vi "LuaTo.vi"(6 "Index":i32, 7 "L In":u64, 8 "Lua Dll":path) -> (0 "String":string, 1 "Variant":variant, 2 "Number":dbl, 3 "Boolean":bool, 4 "L Out":u64, 5 "Pointer":u64)   [LabVIEW 2014]
uses:
  LabVIEW.exe
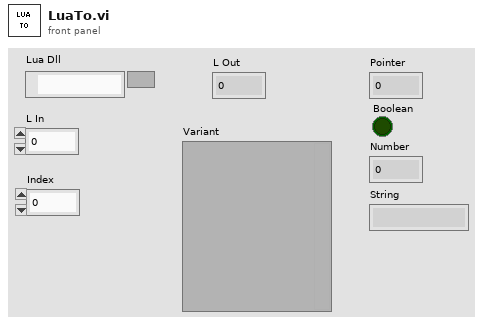
[diagram p1: front panel]
types:
  T1 = enum16{"nil", "boolean", "lightuserdata", "number", "string", "table", "function", "userdata", "thread"}
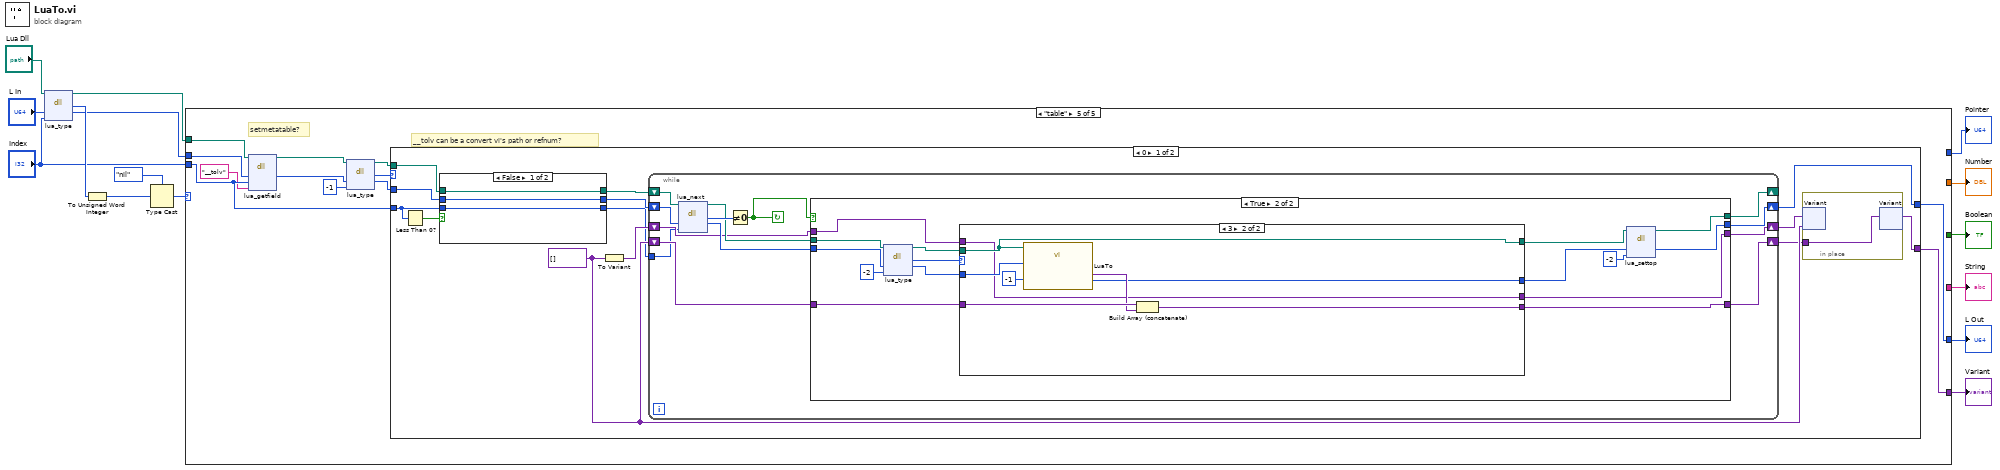
[diagram p0: block diagram]
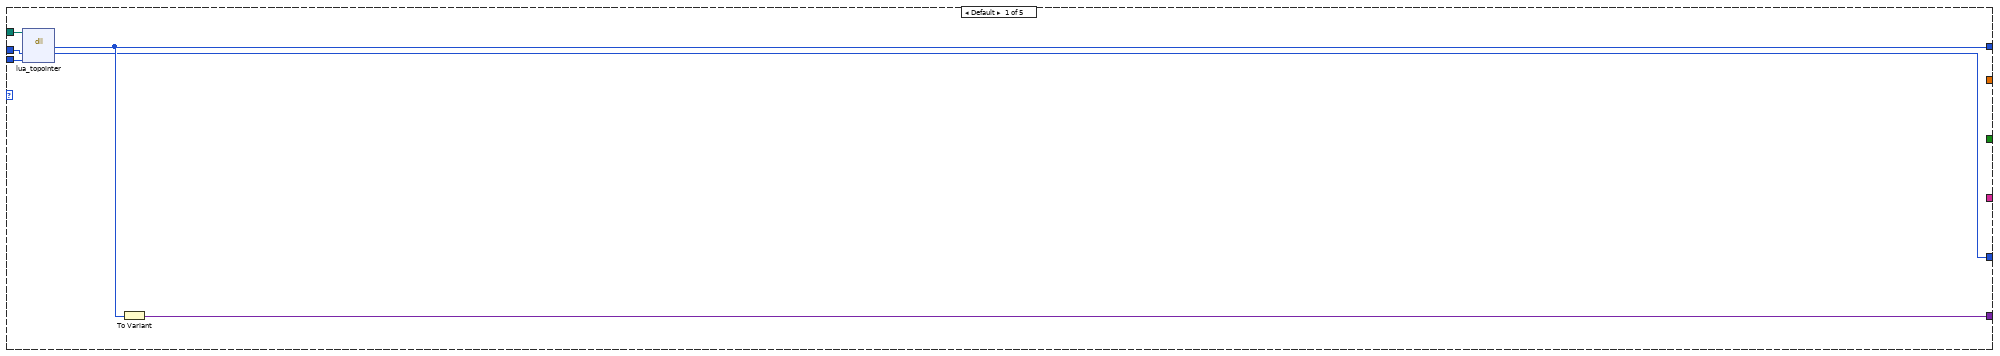
[diagram p2: hidden frame]
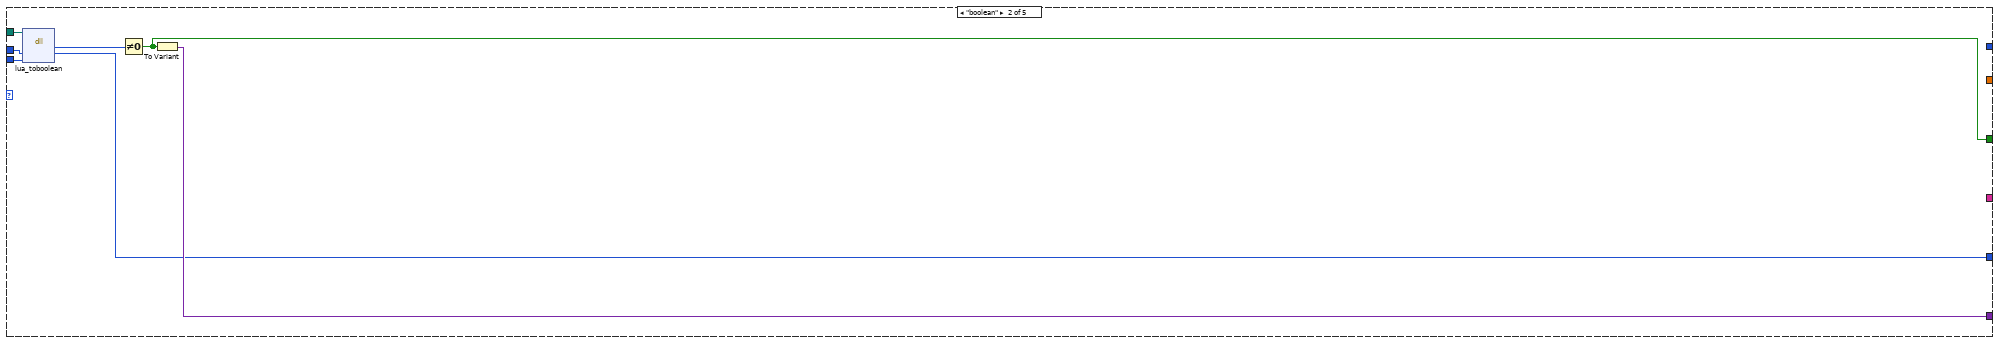
[diagram p3: hidden frame]
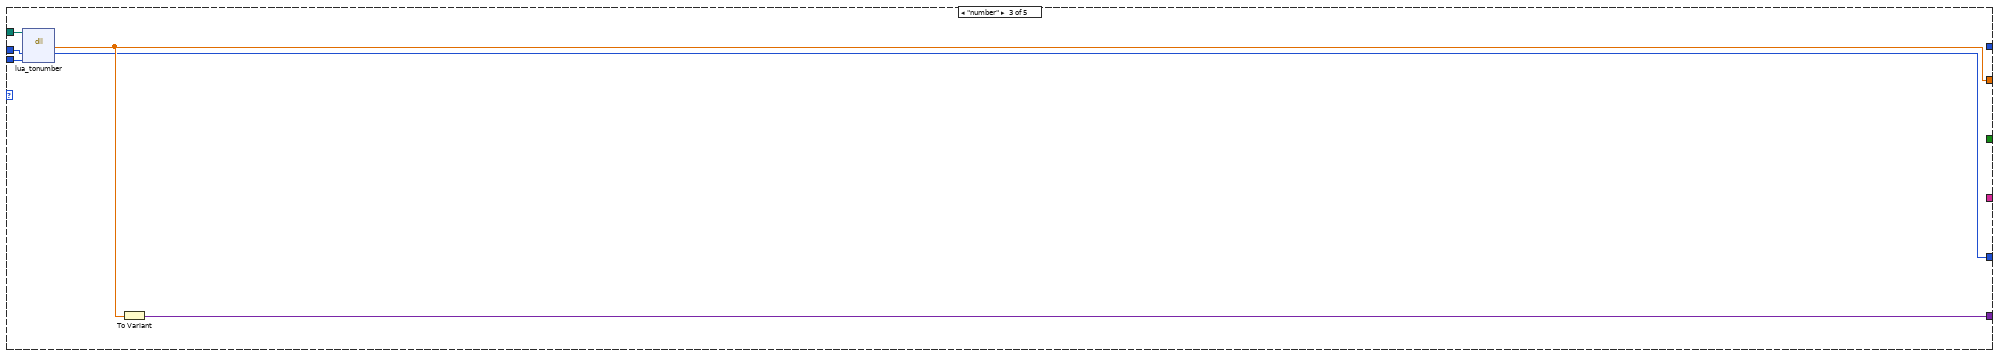
[diagram p4: hidden frame]
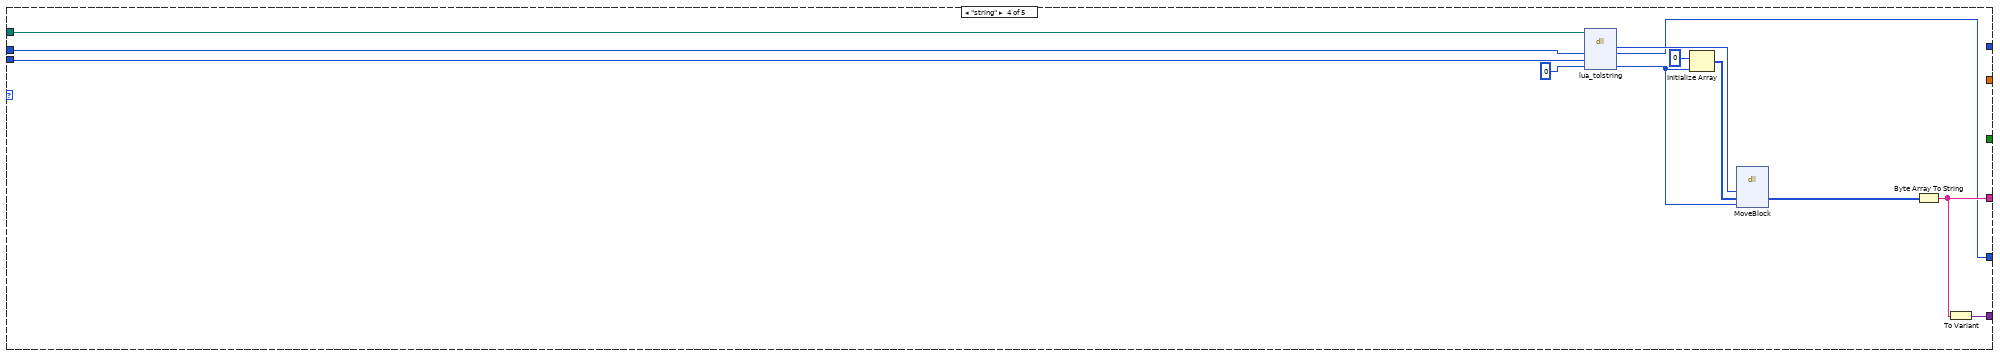
[diagram p5: hidden frame]
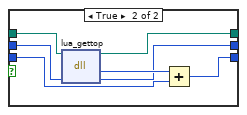
[diagram p6: hidden frame]
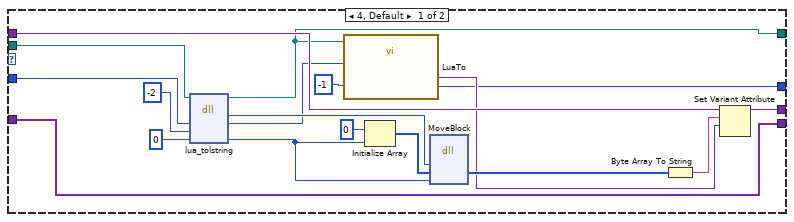
[diagram p8: hidden frame]
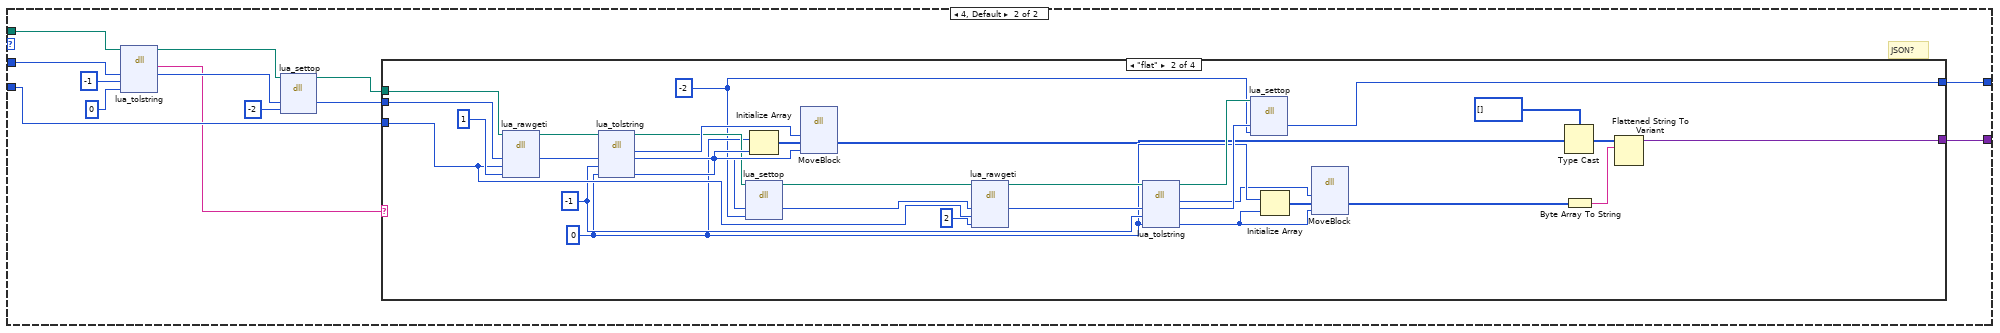
[diagram p9: hidden frame]
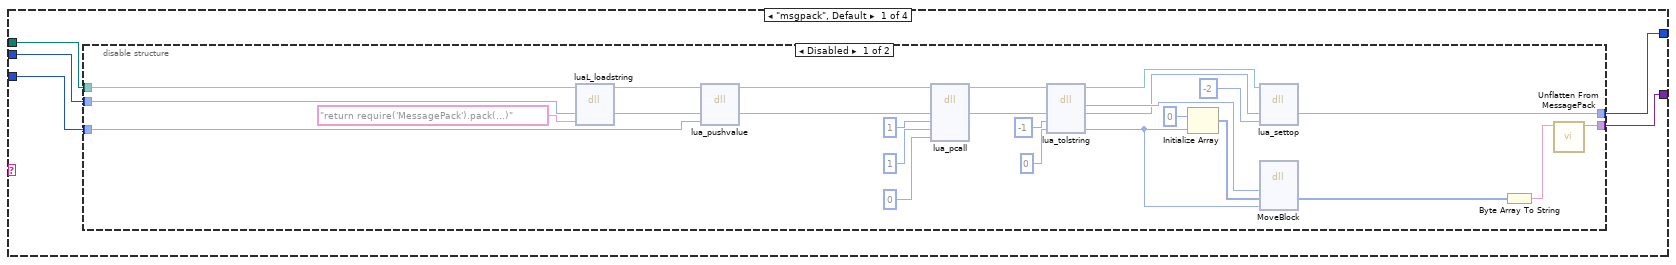
[diagram p10: hidden frame]
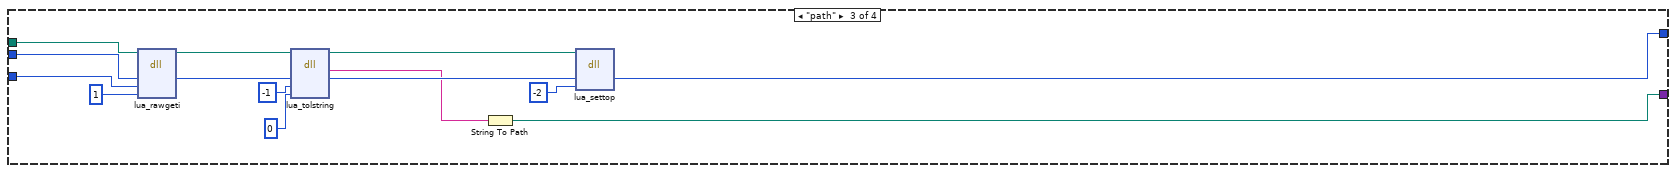
[diagram p12: hidden frame]
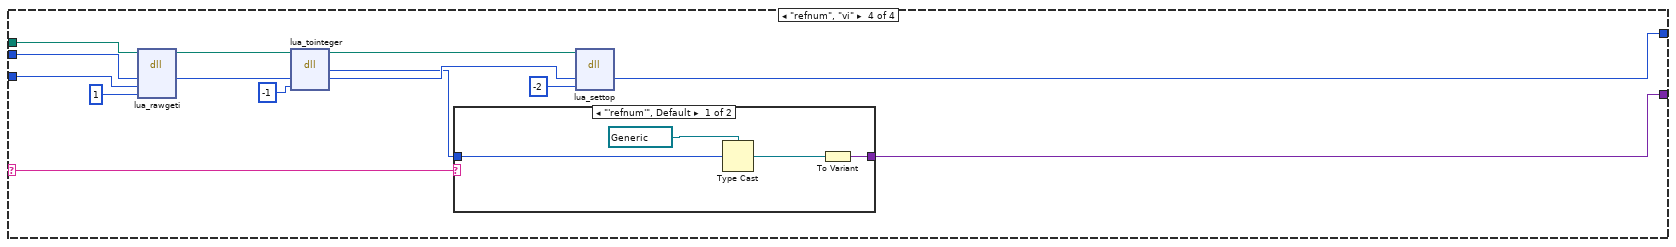
[diagram p13: hidden frame]
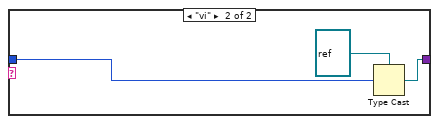
[diagram p14: hidden frame]
diagram:
  n1 = dll-call lib="lua5.dll" fn="lua_type"(path in="Lua Dll", "L"="L In", "idx"="Index") -> (path out=w4:path, "type"=w5:i32, "L"=w3:u64)  [unwired: 3 in, 1 out]
  n2 = To Unsigned Word Integer(number=w5) -> (unsigned 16bit integer=w6:u16)
  n3 = Type Cast(type=T1."nil", x=w6) -> (*(type *) &x=w14:T1)
  n4 = case shown="\"table\"" w14 {
    tunnel: w4 -> [w21 w28 w34 w44 w57]
    tunnel: w3 -> [w20 w27 w33 w43 w56]
    tunnel: [w19 w26 w32 w46 w58] -> w13
    tunnel: [_ w23 _ _ _] -> w9
    tunnel: [w18 _ _ _ _] -> w12
    tunnel: [_ _ w31 _ _] -> w11
    tunnel: "Index" -> [w17 w25 w30 w42 w55]
    tunnel: [_ _ _ w36 _] -> w10
    tunnel: [w16 w22 w29 w35 w47] -> w1
    frame Default {
      n5 = dll-call lib="lua5.dll" fn="lua_topointer"(path in=w21, "L"=w20, "idx"=w17) -> (w18:u64, "L"=w16:u64)  [unwired: 3 in, 2 out]
      n6 = To Variant(anything=w18) -> (Variant=w19:variant)
    }
    frame "boolean" {
      n7 = dll-call lib="lua5.dll" fn="lua_toboolean"(path in=w28, "L"=w27, "idx"=w25) -> (w24:i32, "L"=w22:u64)  [unwired: 3 in, 2 out]
      n8 = Not Equal To 0?(x=w24) -> (x != 0?=w23:bool)
      n9 = To Variant(anything=w23) -> (Variant=w26:variant)
    }
    frame "number" {
      n10 = dll-call lib="lua5.dll" fn="lua_tonumber"(path in=w34, "L"=w33, "idx"=w30) -> (w31:dbl, "L"=w29:u64)  [unwired: 3 in, 2 out]
      n11 = To Variant(anything=w31) -> (Variant=w32:variant)
    }
    frame "string" {
      n12 = dll-call lib="lua5.dll" fn="lua_tolstring"(path in=w44, "L"=w43, "idx"=w42, "len"=0) -> ("str"=w40:u64, "L"=w35:u64, "len"=w38:i32)  [unwired: 3 in, 2 out]
      n13 = Initialize Array(u8 0 ("element"), w38) -> (w39:u8[])
      n14 = dll-call lib="LabVIEW.exe" fn="MoveBlock"("src"=w40, "dest"=w39, "size"=w38) -> ("dest"=w37:u8[])  [unwired: 6 in, 2 out]
      n15 = Byte Array To String(unsigned byte array=w37) -> (string=w36:string)
      n16 = To Variant(anything=w36) -> (Variant=w46:variant)
    }
    frame "table" {
      # "setmetatable?"
      # "__tolv can be a convert vi's path or refnum?"
      n17 = dll-call lib="lua5.dll" fn="lua_getfield"(path in=w57, "L"=w56, "idx"=w55, "name"="__tolv") -> (path out=w53:path, "L"=w51:u64)  [unwired: 5 in, 1 out]
      n18 = dll-call lib="lua5.dll" fn="lua_type"(path in=w53, "L"=w51, "idx"=-1) -> (path out=w52:path, "type"=w48:i32, "L"=w50:u64)  [unwired: 3 in, 1 out]
      n19 = case shown="0" w48 {
        tunnel: w52 -> [w66 w150]
        tunnel: w50 -> [w64 w149]
        tunnel: w55 -> [w60 w153]
        tunnel: [w71 w144] -> w58
        tunnel: [w59 w141] -> w47
        frame 0 {
          w68 = variant[] []
          n20 = Less Than 0?(x=w60) -> (x < 0?=w61:bool)
          n21 = case shown="False" w61 {
            tunnel: w66 -> [w74 w80]
            tunnel: [w74 w79] -> w65
            tunnel: w64 -> [w73 w78]
            tunnel: [w73 w77] -> w63
            tunnel: [w72 w76] -> w62
            tunnel: w60 -> [w72 w75]
            frame False {
            }
            frame True {
              n22 = dll-call lib="lua5.dll" fn="lua_gettop"(path in=w80, "L"=w78) -> (path out=w79:path, w81:i32, "L"=w77:u64)  [unwired: 2 in, 1 out]
              n23 = Add(x=w81, y=w75) -> (x+y=w76:i32)
            }
          }
          n24 = To Variant(anything=w68) -> (Variant=w69:variant)
          n25 = while {
            shift-right: [w85] -> _
            shift-left: w65 -> [w92]
            shift-right: [w84] -> w59
            shift-left: w63 -> [w93]
            shift-right: [w88] -> w67
            shift-left: w68 -> [w89]
            shift-right: [w86] -> w70
            shift-left: w69 -> [w87]
            tunnel: w62 -> [w82]
            stop <- w83 continue-if-true
            n26 = dll-call lib="lua5.dll" fn="lua_next"(path in=w92, "L"=w93, "idx"=w82) -> (path out=w91:path, w94:i32, "L"=w90:u64)  [unwired: 3 in, 1 out]
            n27 = Not Equal To 0?(x=w94) -> (x != 0?=w83:bool)
            n28 = case shown="True" w83 {
              tunnel: w91 -> [w98 w111]
              tunnel: w90 -> [w97 w110]
              tunnel: w89 -> [w95 w105]
              tunnel: [w95 w104] -> w88
              tunnel: w87 -> [w96 w103]
              tunnel: [w96 w102] -> w86
              tunnel: [w98 w101] -> w85
              tunnel: [w97 w100] -> w84
              frame False {
              }
              frame True {
                n29 = dll-call lib="lua5.dll" fn="lua_type"(path in=w111, "L"=w110, "idx"=-2) -> (path out=w107:path, "type"=w108:i32, "L"=w106:u64)  [unwired: 3 in, 1 out]
                n30 = case shown="3" w108 {
                  tunnel: w107 -> [w131 w135]
                  tunnel: w106 -> [w130 w134]
                  tunnel: w105 -> [w127 w138]
                  tunnel: [w127 w136] -> w104
                  tunnel: [w118 w135] -> w113
                  tunnel: [w114 w132] -> w112
                  tunnel: w103 -> [w129 w133]
                  tunnel: [w128 w133] -> w102
                  frame 4, Default {
                    n31 = dll-call lib="lua5.dll" fn="lua_tolstring"(path in=w131, "L"=w130, "idx"=-2, "len"=0) -> (path out=w118:path, "str"=w123:u64, "L"=w117:u64, "len"=w121:i32)  [unwired: 3 in, 1 out]
                    n32 = call "LuaTo.vi"("Index"=-1 ("n"), "L In"=w117, "Lua Dll"=w118) -> ("Variant"=w115:variant, "L Out"=w114:u64)  [unwired: 4 out]
                    n33 = Initialize Array(u8 0 ("element"), w121) -> (w122:u8[])
                    n34 = dll-call lib="LabVIEW.exe" fn="MoveBlock"("src"=w123, "dest"=w122, "size"=w121) -> ("dest"=w119:u8[])  [unwired: 6 in, 2 out]
                    n35 = Byte Array To String(unsigned byte array=w119) -> (string=w126:string)
                    n36 = Set Variant Attribute(Variant=w129, name=w126, value=w115) -> (Variant out=w128:variant)  [unwired: 1 in, 2 out]
                  }
                  frame 3 {
                    n37 = call "LuaTo.vi"("Index"=-1 ("n"), "L In"=w134, "Lua Dll"=w135) -> ("Variant"=w137:variant, "L Out"=w132:u64)  [unwired: 4 out]
                    n38 = Build Array (concatenate)(w138, w137) -> (w136:variant[])
                  }
                }
                n39 = dll-call lib="lua5.dll" fn="lua_settop"(path in=w113, "L"=w112, "idx"=-2) -> (path out=w101:path, "L"=w100:u64)  [unwired: 4 in, 1 out]
              }
            }
          }
          n40 = in-place {
            in-place-border: w67 -> [w140]
            n41 = in-place-variant #1(w70, w68) -> ()  [unwired: 2 out]
            n42 = in-place-variant #1(w140) -> (w71:variant)  [unwired: 1 out]
          }
        }
        frame 4, Default {
          # "JSON?"
          n43 = dll-call lib="lua5.dll" fn="lua_tolstring"(path in=w150, "L"=w149, "idx"=-1, "len"=0) -> (path out=w152:path, "str"=w143:string, "L"=w145:u64)  [unwired: 4 in, 1 out]
          n44 = dll-call lib="lua5.dll" fn="lua_settop"(path in=w152, "L"=w145, "idx"=-2) -> (path out=w151:path, "L"=w148:u64)  [unwired: 4 in, 1 out]
          n45 = case shown="\"flat\"" w143 {
            selector: w143 -> [_ _ _ w232]
            tunnel: w153 -> [w158 w206 w224 w242]
            tunnel: w151 -> [w157 w216 w230 w244]
            tunnel: w148 -> [w156 w215 w227 w243]
            tunnel: [w155 w188 w218 w233] -> w144
            tunnel: [w154 w186 w217 w231] -> w141
            frame "msgpack", Default {
              n46 = disable-structure shown="Disabled" {
                disable-tunnel: w158 -> [w163 _]
                disable-tunnel: w157 -> [w162 _]
                disable-tunnel: w156 -> [w161 w185]
                disable-tunnel: [w160 _] -> w155
                disable-tunnel: [w159 w185] -> w154
                frame Disabled {
                  n47 = dll-call lib="lua5.dll" fn="luaL_loadstring"(path in=w162, "L"=w161, "str"="return require('MessagePack').pack(...)") -> (path out=w178:path, "L"=w176:u64)  [unwired: 4 in, 1 out]
                  n48 = dll-call lib="lua5.dll" fn="lua_pushvalue"(path in=w178, "L"=w176, "idx"=w163) -> (path out=w177:path, "L"=w175:u64)  [unwired: 4 in, 1 out]
                  n49 = dll-call lib="lua5.dll" fn="lua_pcall"(path in=w177, "L"=w175, "nargs"=1, "nresults"=1, "errfunc"=0) -> (path out=w184:path, "L"=w183:u64)  [unwired: 6 in, 1 out]
                  n50 = dll-call lib="lua5.dll" fn="lua_tolstring"(path in=w184, "L"=w183, "idx"=-1, "len"=0) -> (path out=w165:path, "str"=w172:u64, "L"=w166:u64, "len"=w170:i32)  [unwired: 3 in, 1 out]
                  n51 = Initialize Array(u8 0 ("element"), w170) -> (w171:u8[])
                  n52 = dll-call lib="lua5.dll" fn="lua_settop"(path in=w165, "L"=w166, "idx"=-2) -> ("L"=w159:u64)  [unwired: 4 in, 2 out]
                  n53 = dll-call lib="LabVIEW.exe" fn="MoveBlock"("src"=w172, "dest"=w171, "size"=w170) -> ("dest"=w169:u8[])  [unwired: 6 in, 2 out]
                  n54 = Byte Array To String(unsigned byte array=w169) -> (string=w167:string)
                  n55 = call "Unflatten From MessagePack.vi"("MsgPack Data"=w167) -> ("Data"=w160:variant)  [unwired: 9 in, 1 out]
                }
                frame Enabled {
                }
              }
            }
            frame "flat" {
              w187 = -2 ("idx")
              w197 = 0 ("len")
              w198 = -1 ("idx")
              n56 = dll-call lib="lua5.dll" fn="lua_rawgeti"(path in=w216, "L"=w215, "idx"=w206, "i"=1) -> (path out=w213:path, "L"=w212:u64)  [unwired: 5 in, 1 out]
              n57 = dll-call lib="lua5.dll" fn="lua_tolstring"(path in=w213, "L"=w212, "idx"=w198, "len"=w197) -> (path out=w204:path, "str"=w210:u64, "L"=w202:u64, "len"=w209:i32)  [unwired: 3 in, 1 out]
              n58 = dll-call lib="lua5.dll" fn="lua_settop"(path in=w204, "L"=w202, "idx"=w187) -> (path out=w203:path, "L"=w201:u64)  [unwired: 4 in, 1 out]
              n59 = Initialize Array(w197, w209) -> (w211:i32[])
              n60 = dll-call lib="LabVIEW.exe" fn="MoveBlock"("src"=w210, "dest"=w211, "size"=w209) -> ("dest"=w189:u8[])  [unwired: 6 in, 2 out]
              n61 = dll-call lib="lua5.dll" fn="lua_rawgeti"(path in=w203, "L"=w201, "idx"=w206, "i"=2) -> (path out=w208:path, "L"=w207:u64)  [unwired: 5 in, 1 out]
              n62 = dll-call lib="lua5.dll" fn="lua_tolstring"(path in=w208, "L"=w207, "idx"=w198, "len"=w197) -> (path out=w199:path, "str"=w195:u64, "L"=w200:u64, "len"=w194:i32)  [unwired: 3 in, 1 out]
              n63 = dll-call lib="lua5.dll" fn="lua_settop"(path in=w199, "L"=w200, "idx"=w187) -> ("L"=w186:u64)  [unwired: 4 in, 2 out]
              n64 = Initialize Array(w197, w194) -> (w196:i32[])
              n65 = dll-call lib="LabVIEW.exe" fn="MoveBlock"("src"=w195, "dest"=w196, "size"=w194) -> ("dest"=w193:u8[])  [unwired: 6 in, 2 out]
              n66 = Type Cast(type=i16[] [] ("type string"), x=w189) -> (*(type *) &x=w190:i16[])
              n67 = Byte Array To String(unsigned byte array=w193) -> (string=w192:string)
              n68 = Flattened String To Variant(6:w192, 7:w190) -> (3:w188:variant)  [unwired: 1 in, 1 out]
            }
            frame "path" {
              n69 = dll-call lib="lua5.dll" fn="lua_rawgeti"(path in=w230, "L"=w227, "idx"=w224, "i"=1) -> (path out=w229:path, "L"=w226:u64)  [unwired: 5 in, 1 out]
              n70 = dll-call lib="lua5.dll" fn="lua_tolstring"(path in=w229, "L"=w226, "idx"=-1, "len"=0) -> (path out=w228:path, "str"=w219:string, "L"=w225:u64)  [unwired: 4 in, 1 out]
              n71 = String To Path(string=w219) -> (path=w218:path)
              n72 = dll-call lib="lua5.dll" fn="lua_settop"(path in=w228, "L"=w225, "idx"=-2) -> ("L"=w217:u64)  [unwired: 4 in, 2 out]
            }
            frame "refnum", "vi" {
              n73 = dll-call lib="lua5.dll" fn="lua_rawgeti"(path in=w244, "L"=w243, "idx"=w242, "i"=1) -> (path out=w239:path, "L"=w240:u64)  [unwired: 5 in, 1 out]
              n74 = dll-call lib="lua5.dll" fn="lua_tointeger"(path in=w239, "L"=w240, "idx"=-1) -> (path out=w236:path, w234:u32, "L"=w235:u64)  [unwired: 3 in, 1 out]
              n75 = case shown="\"'refnum'\", Default" w232 {
                tunnel: w234 -> [w247 w251]
                tunnel: [w245 w249] -> w233
                frame "'refnum'", Default {
                  n76 = Type Cast(type=refnum<vi> refnum ("reference"), x=w247) -> (*(type *) &x=w246:refnum<vi>)
                  n77 = To Variant(anything=w246) -> (Variant=w245:variant)
                }
                frame "vi" {
                  n78 = Type Cast(type=refnum<vi> refnum ("vi reference"), x=w251) -> (*(type *) &x=w249:refnum<vi>)
                }
              }
              n79 = dll-call lib="lua5.dll" fn="lua_settop"(path in=w236, "L"=w235, "idx"=-2) -> ("L"=w231:u64)  [unwired: 4 in, 2 out]
            }
          }
        }
      }
    }
  }
  "Variant" <- w13
  "Pointer" <- w12
  "Number" <- w11
  "String" <- w10
  "Boolean" <- w9
  "L Out" <- w1
